vi "LogCanRxMessage.vi"(0 "GenericCanAdapterClass in":refnum<class "GenericCanAdapterClass.lvclass">, 1 "LogSuspend":bool, 5 "Arbitration Id":u32 format="%08x", 7 "DataLength":u16, 9 "Data":u8[](array[numeric]) format="%02x", 11 "error in":errorcluster) -> (4 "GenericCanAdapterClass out":refnum<class "GenericCanAdapterClass.lvclass">, 15 "error out":errorcluster)   [LabVIEW 2011, in "GenericCanAdapterClass.lvclass"]
uses:
  GenericCanAdapterClass.lvclass
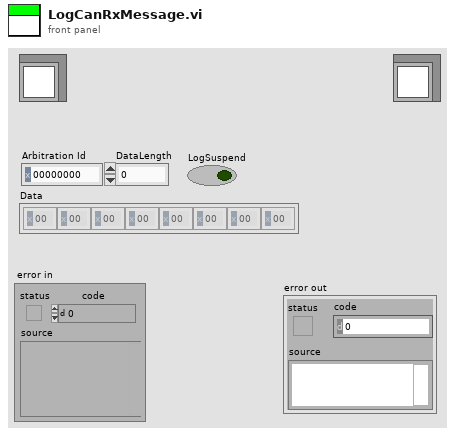
[diagram p1: front panel]
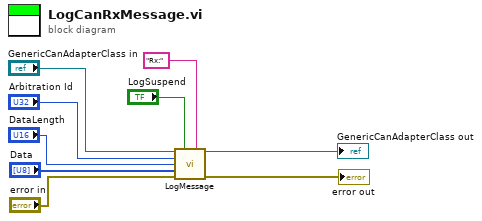
[diagram p0: block diagram]
diagram:
  n1 = call "LogMessage.vi"("GenericCanAdapterClass in"="GenericCanAdapterClass in", "LogSuspend"="LogSuspend", "Name"="Rx:", "Arbitration Id"="Arbitration Id", "DataLength"="DataLength", "Data"="Data", "error in"="error in") -> ("GenericCanAdapterClass out"=→"GenericCanAdapterClass out":refnum<class "GenericCanAdapterClass.lvclass">, "error out"=→"error out":errorcluster)  [unwired: 7 in]
